vi "Plot Editor_Controls to Store.vi"(8 "Error In":errorcluster, 10 "Control Refnums":refnum<vi>[](array[refnum]), 11 "Plot Editor Internal Data in":T1) -> (0 "Error Out":errorcluster, 3 "Plot Editor Internal Data out":T1)   [LabVIEW 2019, in "Plot Editor.lvlib"]
uses:
  Plot Editor.lvlib
  Plot Editor Internal Variables.ctl
  XY Graph Plot Properties.ctl
panel:
  in  "Array":refnum<vi>
  in  "Numeric":refnum<vi>
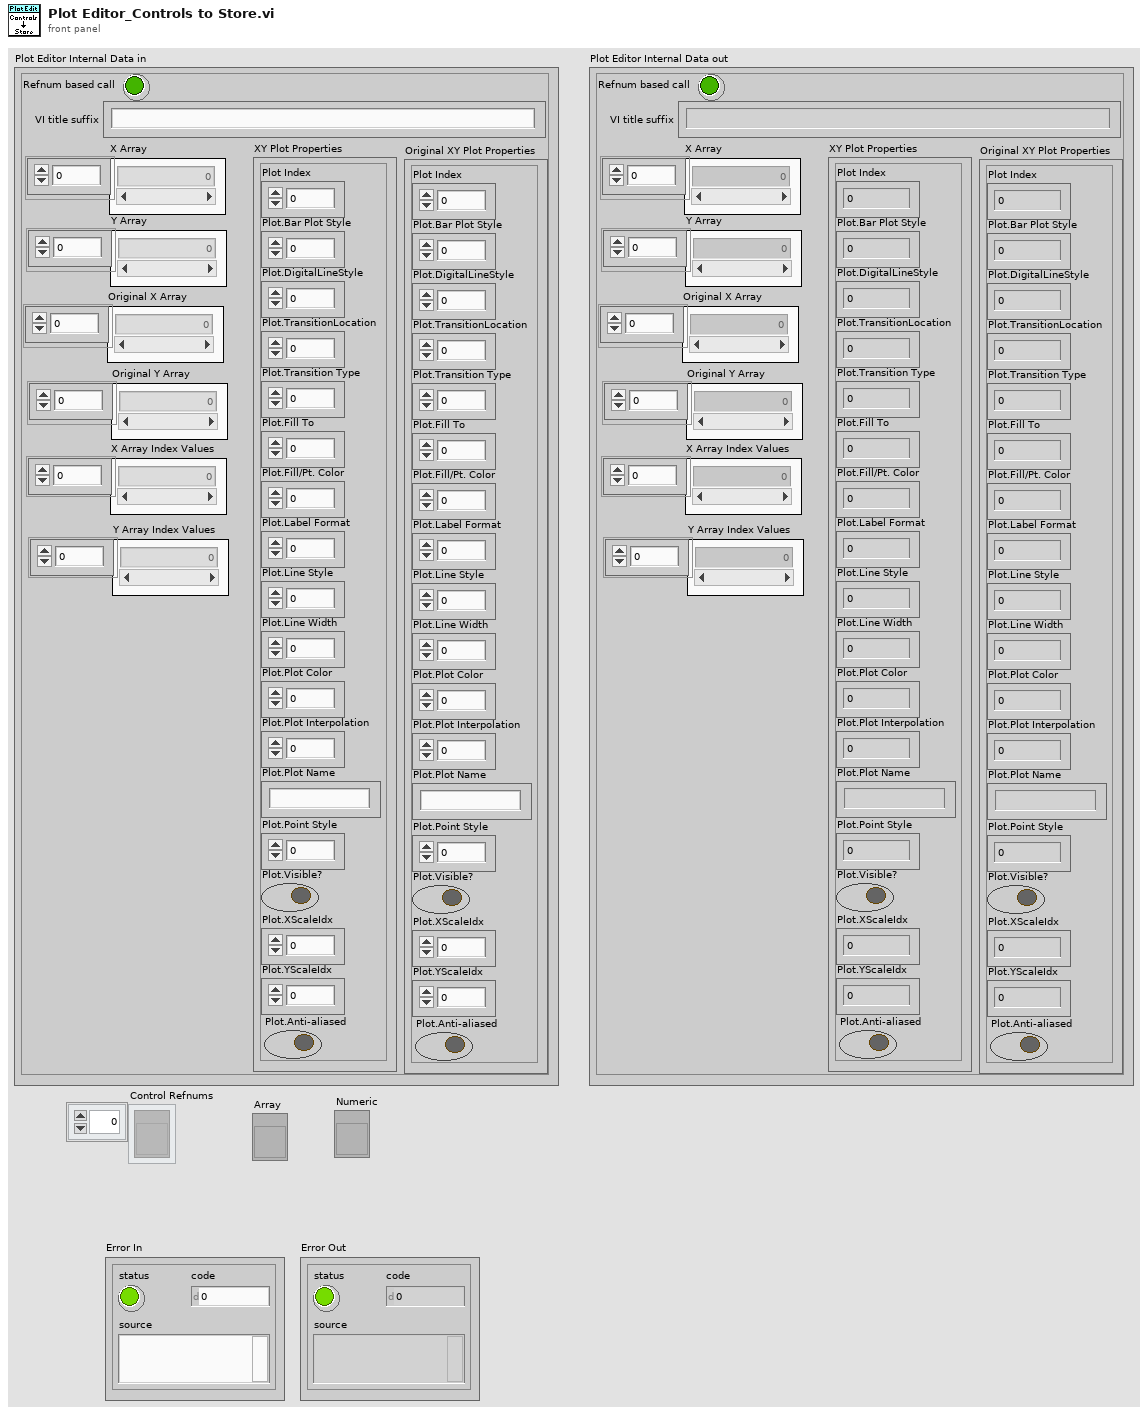
[diagram p1: front panel]
types:
  T1 = typedef "Plot Editor.lvlib/Plot Editor Internal Variables.ctl" = cluster{"X Array":dbl[], "Y Array":dbl[], "XY Plot Properties":T2, "X Array Index Values":u32[], "Y Array Index Values":u32[], "Original XY Plot Properties":T2, "Original X Array":dbl[], "Original Y Array":dbl[], "VI title suffix":string, "Refnum based call":bool}
  T2 = typedef "XY Graph Plot Properties.ctl" = cluster{"Plot Index":i32, "Plot.Bar Plot Style":u8, "Plot.DigitalLineStyle":u8, "Plot.TransitionLocation":u8, "Plot.Transition Type":u8, "Plot.Fill To":i16, "Plot.Fill/Pt. Color":u32, "Plot.Label Format":u8, "Plot.Line Style":u8, "Plot.Line Width":u8, "Plot.Plot Color":u32, "Plot.Plot Interpolation":u8, "Plot.Plot Name":string, "Plot.Point Style":u8, "Plot.Visible?":bool, "Plot.XScaleIdx":u32, "Plot.YScaleIdx":u32, "Plot.Anti-aliased":bool}
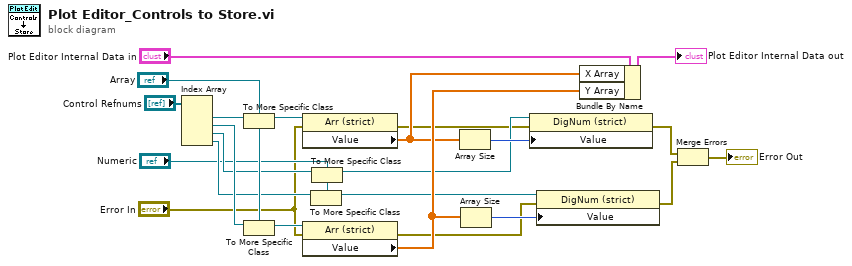
[diagram p0: block diagram]
diagram:
  n1 = Index Array(array="Control Refnums") -> (element #1=w16:refnum<vi>, element #2=w14:refnum<vi>, element #3=w11:refnum<vi>, element #4=w9:refnum<vi>)  [unwired: 4 in]
  n2 = To More Specific Class(target class="Array", reference=w16) -> (specific class reference=w15:refnum<vi>)  [unwired: 1 in, 1 out]
  n3 = To More Specific Class(target class="Array", reference=w14) -> (specific class reference=w12:refnum<vi>)  [unwired: 1 in, 1 out]
  n4 = property class="Arr (strict)"(reference=w15, error in="Error In") -> (error out=w5:errorcluster, "Value"=w22:dbl[])  [unwired: 1 out]
  n5 = property class="Arr (strict)"(reference=w12, error in="Error In") -> (error out=w4:errorcluster, "Value"=w23:dbl[])  [unwired: 1 out]
  n6 = To More Specific Class(target class="Numeric", reference=w9) -> (specific class reference=w7:refnum<vi>)  [unwired: 1 in, 1 out]
  n7 = To More Specific Class(target class="Numeric", reference=w11) -> (specific class reference=w10:refnum<vi>)  [unwired: 1 in, 1 out]
  n8 = Array Size(array=w22) -> (size(s)=w20:i32)
  n9 = Array Size(array=w23) -> (size(s)=w21:i32)
  n10 = property class="DigNum (strict)"(reference=w10, error in=w5, "Value"=w20) -> (error out=w3:errorcluster)  [unwired: 1 out]
  n11 = property class="DigNum (strict)"(reference=w7, error in=w4, "Value"=w21) -> (error out=w1:errorcluster)  [unwired: 1 out]
  n12 = Bundle By Name(cluster="Plot Editor Internal Data in", "X Array"=w22, "Y Array"=w23) -> (→"Plot Editor Internal Data out":T1)
  n13 = Merge Errors(w3, w1) -> (→"Error Out":errorcluster)
